vi "Request and Send Data.vi"(8 "error in":errorcluster, 11 "DAQ Device in":refnum<class "DAQ Device.lvclass">) -> (0 "error out":errorcluster, 3 "DAQ Device out":refnum<class "DAQ Device.lvclass">)   [LabVIEW 2014, in "DAQ Device.lvclass"]
uses:
  DAQ Device.lvclass
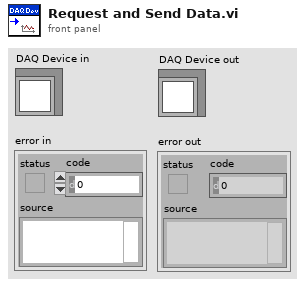
[diagram p1: front panel]
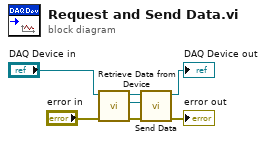
[diagram p0: block diagram]
diagram:
  n1 = call-dynamic "Retrieve Data from Device.vi"("error in (no error)"="error in", "DAQ Device in"="DAQ Device in") -> ("error out"=w3:errorcluster, "Data"=w2:refnum<class "Data.lvclass">, "DAQ Device out"=w6:refnum<class "DAQ Device.lvclass">)  [unwired: 7 in]
  n2 = call-dynamic "Send Data.vi"("error in"=w3, "Data"=w2, "DAQ Device in"=w6) -> ("error out"=→"error out":errorcluster, "DAQ Device out"=→"DAQ Device out":refnum<class "DAQ Device.lvclass">)  [unwired: 7 in]
